vi "timer (SubVI).vi"(8 "error in (no error)":errorcluster, 11 "Action":T1) -> (0 "error out":errorcluster, 3 "Numeric":u32)   [LabVIEW 2023]
doc: "Deafult timer, with 3 actions, reset, pause and run. Return time elapsed from last reset."
uses:
  #typedef_action.ctl
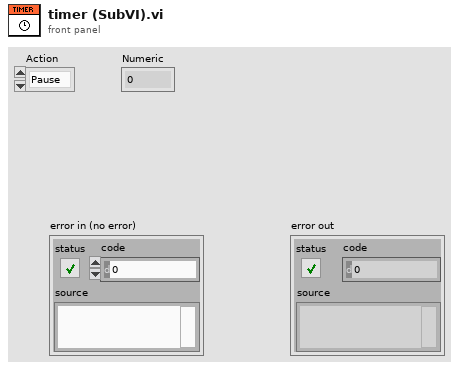
[diagram p1: front panel]
types:
  T1 = typedef "#typedef_action.ctl" = enum16{"Pause", "Reset", "Run"}
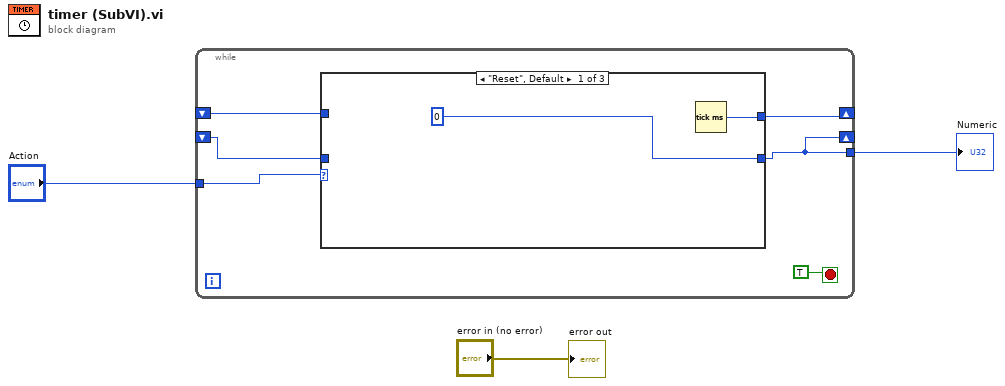
[diagram p0: block diagram]
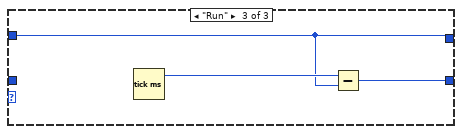
[diagram p3: hidden frame]
diagram:
  n1 = while {
    shift-right: [w8] -> _
    shift-left: _ -> [w7]
    tunnel: "Action" -> [w9]
    tunnel: [w5] -> w2
    shift-right: [w5] -> _
    shift-left: _ -> [w4]
    stop <- TRUE stop-if-true
    n2 = case shown="\"Reset\", Default" w9 {
      tunnel: [w10 w13 w15] -> w8
      tunnel: w7 -> [_ w13 w15]
      tunnel: [0 w12 w14] -> w5
      tunnel: w4 -> [_ w12 _]
      frame "Reset", Default {
        n3 = Tick Count (ms)() -> (millisecond timer value=w10:u32)
      }
      frame "Pause" {
      }
      frame "Run" {
        n4 = Tick Count (ms)() -> (millisecond timer value=w16:u32)
        n5 = Subtract(x=w16, y=w15) -> (x-y=w14:u32)
      }
    }
  }
  "Numeric" <- w2
  "error out" <- "error in (no error)"
